vi "Write SA Pin.vi"(8 "error in (no error)":errorcluster, 10 "SA Pin":string, 11 "CDMA2K_CHP in":refnum<class "CDMA2K_CHP.lvclass">=refnum) -> (0 "error out":errorcluster, 3 "CDMA2K_CHP out":refnum<class "CDMA2K_CHP.lvclass">)   [LabVIEW 2016, in "SeqAuto Evaluations.lvlib" / "CDMA2K_CHP.lvclass"]
uses:
  CDMA2K_CHP.lvclass
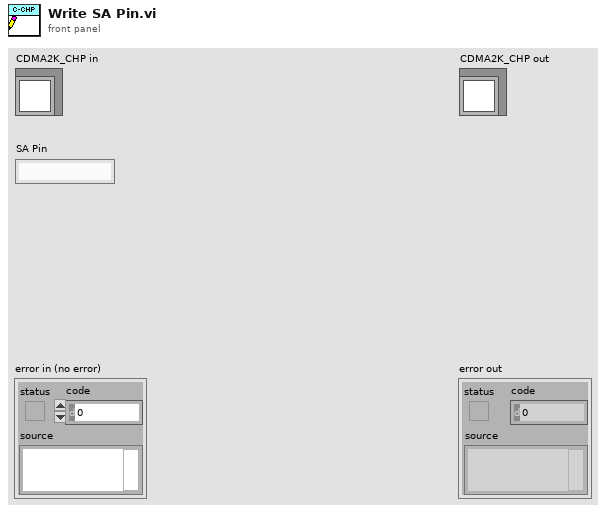
[diagram p1: front panel]
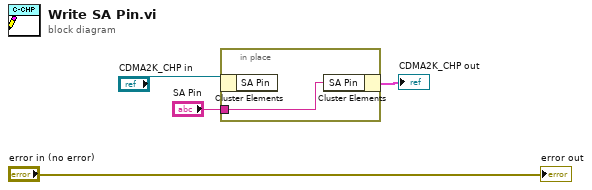
[diagram p0: block diagram]
diagram:
  n1 = in-place {
    in-place-border: "SA Pin" -> [w5]
    n2 = in-place-cluster #1("CDMA2K_CHP in") -> ()  [unwired: 1 out]
    n3 = in-place-cluster #1("SA Pin"=w5) -> (→"CDMA2K_CHP out":cluster{})
  }
  "error out" <- "error in (no error)"
